vi "MinusPlus.vi"(10 "Wrap":i32, 11 "Index":i32) -> (2 "Plus":i32, 3 "Minus":i32)   [LabVIEW 2014]
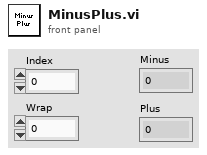
[diagram p1: front panel]
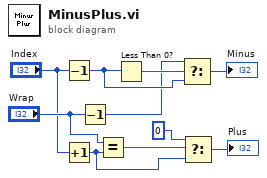
[diagram p0: block diagram]
diagram:
  n1 = Decrement(x="Index") -> (x-1=w9:i32)
  n2 = Increment(x="Index") -> (x+1=w1:i32)
  n3 = Decrement(x="Wrap") -> (x-1=w7:i32)
  n4 = Equal?(x="Wrap", y=w1) -> (x = y?=w5:bool)
  n5 = Less Than 0?(x=w9) -> (x < 0?=w10:bool)
  n6 = Select(t=w7, s=w10, f=w9) -> (s? t:f=→"Minus":i32)
  n7 = Select(t=0, s=w5, f=w1) -> (s? t:f=→"Plus":i32)
